vi "6509_init.vi"(8 "error in":errorcluster, 9 "sample mode":i32(ring)=10123 items=["Finite Samples"=10178, "Continuous Samples"=10123, "Hardware Timed Single Point"=12522], 10 "line grouping":i32(ring)=1 items=["one channel for each line", "one channel for all lines"], 11 "lines in":tag="Dev1/port8/line6:7") -> (0 "error out":errorcluster, 2 "signalType":i32(ring)=12530 items=["Sample Complete Event"=12530, "Counter Output Event"=12494, "Change Detection Event"=12511, "Sample Clock"=12487], 3 "task out":refnum<k21>)   [LabVIEW 2018, in "6509.lvlib"]
uses:
  Libraries/6509/6509.lvlib
  <vilib>/DAQmx/create/channels.llb/DAQmx Create Channel (DI-Digital Input).vi
  <vilib>/DAQmx/configure/timing.llb/DAQmx Timing (Change Detection).vi
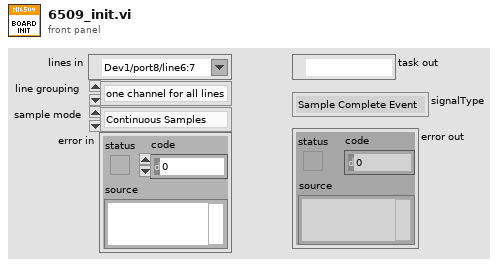
[diagram p1: front panel]
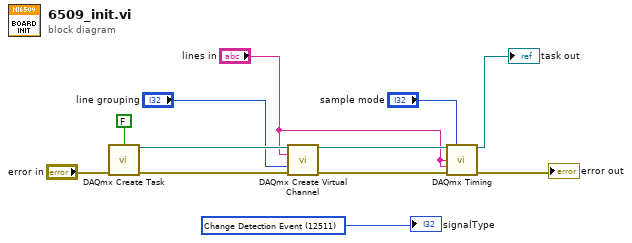
[diagram p0: block diagram]
diagram:
  w1 = 12511 items=["Sample Complete Event"=12530, "Counter Output Event"=12494, "Change Detection Event"=12511, "Sample Clock"=12487] ("signalType")
  n1 = call <vilib>:"DAQmx Create Task.vi"("auto cleanup"=FALSE, "error in"="error in") -> ("task out"=w10:refnum<k21>, "error out"=w8:errorcluster)  [unwired: 12 in]
  n2 = call-poly <vilib>:"DAQmx Create Virtual Channel.vi"("task in"=w10, "lines"="lines in", "line grouping"="line grouping", "error in"=w8) -> ("task out"=w12:refnum<k21>, "error out"=w11:errorcluster)  [unwired: 10 in]
  n3 = call-poly <vilib>:"DAQmx Timing.vi"("task/channels in"=w12, "sample mode"="sample mode", "rising edge physical channels"="lines in", "falling edge physical channels"="lines in", "error in"=w11) -> ("task out"=→"task out":refnum<k21>, "error out"=→"error out":errorcluster)  [unwired: 9 in]
  "signalType" <- w1
